vi "DeleteAll.vi"(8 "error":errorcluster caption="错误输入（无错误）", 11 "Excel._Worksheet":refnum<k7>) -> (0 "error out":errorcluster caption="错误输出", 3 "Excel._Worksheet":refnum<k7>)   [LabVIEW 2014]
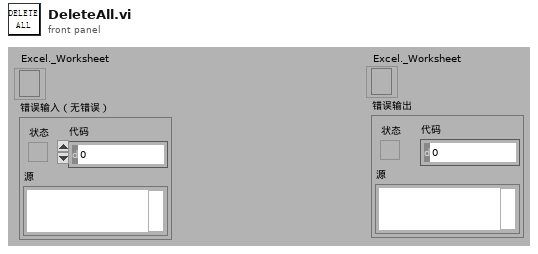
[diagram p1: front panel]
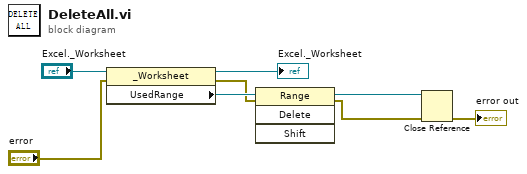
[diagram p0: block diagram]
diagram:
  n1 = property class="_Worksheet"(reference="Excel._Worksheet", error in="error") -> (reference out=→"Excel._Worksheet":refnum<k7>, error out=w1:errorcluster, "UsedRange"=w2:refnum<k7>)
  n2 = invoke class="Range" method="Delete"(reference=w2, error in=w1) -> (reference out=w8:refnum<k7>, error out=w3:errorcluster)  [unwired: 2 in, 2 out]
  n3 = Close Reference(reference=w8, error in (no error)=w3) -> (error out=→"error out":errorcluster)
